vi "Publish Line Control.vi"(8 "error in (no error)":errorcluster, 10 "Status (Out Of Range)":T1=enum."Out of range", 11 "Sample Line in":refnum<class "Sample Line.lvclass">) -> (0 "error out":errorcluster, 3 "Sample Line out":refnum<class "Sample Line.lvclass">)   [LabVIEW 2015, in "cRIO-Carbondioxide.lvlib" / "CO2-Actor.lvlib" / "Sample Line.lvclass"]
uses:
  Sample Line.lvclass
  Controls/Sample Line State Enumerator.ctl
  Sample Line.lvclass/Sample Line.ctl
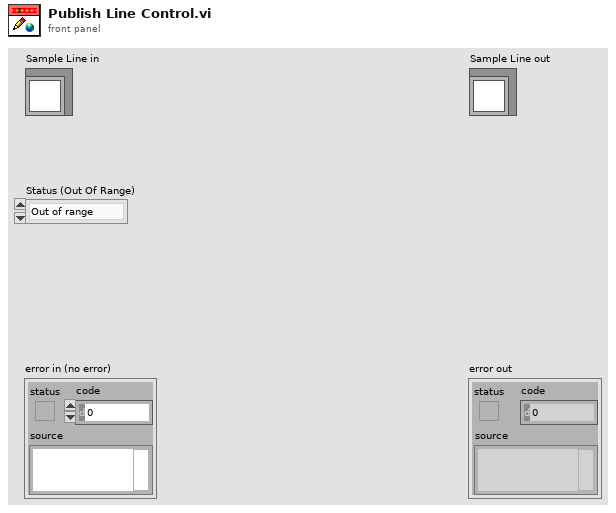
[diagram p1: front panel]
types:
  T1 = typedef "Sample Line State Enumerator.ctl" = enum16{"All lines closed", "Sample line 1.", "Sample line 2.", "Sample line 3.", "Sample line 4.", "Sample line 5.", "Out of range"}
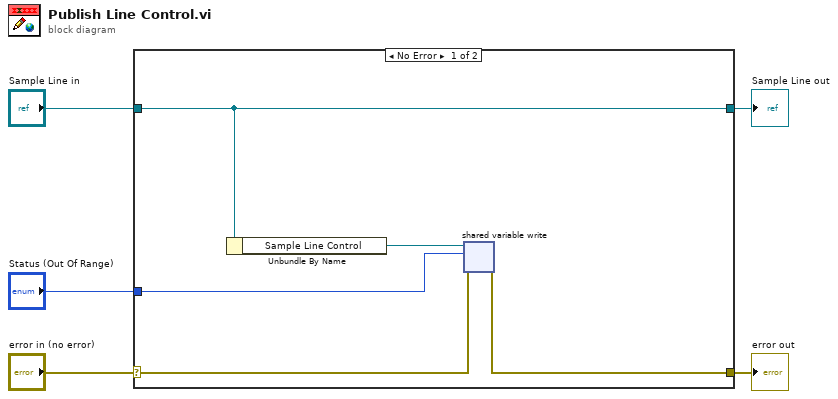
[diagram p0: block diagram]
diagram:
  n1 = case shown="No Error" "error in (no error)" {
    selector: "error in (no error)" -> [w8 w12]
    tunnel: [w7 w12] -> w4
    tunnel: [w10 w11] -> w2
    tunnel: "Sample Line in" -> [w10 w11]
    tunnel: "Status (Out Of Range)" -> [w6 _]
    frame No Error {
      n2 = Unbundle By Name(w10) -> ("Sample Line Control"=w9:refnum<k21>)
      n3 = shared-variable-write(w9, w8, w6) -> (w7:errorcluster)  [unwired: 1 out]
    }
    frame Error {
    }
  }
  "error out" <- w4
  "Sample Line out" <- w2
